vi "Post Initialize Action.vi"(8 "error in (no error)":errorcluster, 11 "Main Window in":refnum<class "Main Window.lvclass">) -> (0 "error out":errorcluster, 2 "Init Event Data":variant, 3 "Main Window out":refnum<class "Main Window.lvclass">)   [LabVIEW 2021, in "Recipe.lvlib" / "Main Window.lvclass"]
doc: "This VI is called just after the Panel Actor's UI was initialized.\n\nData wired to <b>Init Event Data</b> will be passed in the panel's \"Initialized\" user event.\n\nIf there were any initialization errors they should be handled here.\n\n----\nPlease see the following web address for additional documentation and tutorial information:\nhttp://www.mooregoodideas.com/mgi-panel-manager/\n\nAuthor: Derek Trepanier\n\nCopyright (c) 2018, Moore Good Ideas, Inc.\n\nAll rights reserved.\n\nRedistribution and use in source and binary forms, with or without modification, are permitted provided that the following conditions are met:\n\n * Redistributions of source code must retain the above copyright notice, this list of conditions and the following disclaimer.\n * Redistributions in binary form must reproduce the above copyright notice, this list of conditions and the following disclaimer in the documentation and/or other materials provided with the distribution.\n * Neither the name of Moore Good Ideas, Inc. nor the names of its contributors may be used to endorse or promote products derived from this software without specific prior written permission.\n\nTHIS SOFTWARE IS PROVIDED BY THE COPYRIGHT HOLDERS AND CONTRIBUTORS \"AS IS\" AND ANY EXPRESS OR IMPLIED WARRANTIES, INCLUDING, BUT NOT LIMITED TO, THE IMPLIED WARRANTIES OF MERCHANTABILITY AND FITNESS FOR A PARTICULAR PURPOSE ARE DISCLAIMED. IN NO EVENT SHALL THE COPYRIGHT OWNER OR CONTRIBUTORS BE LIABLE FOR ANY DIRECT, INDIRECT, INCIDENTAL, SPECIAL, EXEMPLARY, OR CONSEQUENTIAL DAMAGES (INCLUDING, BUT NOT LIMITED TO, PROCUREMENT OF SUBSTITUTE GOODS OR SERVICES; LOSS OF USE, DATA, OR PROFITS; OR BUSINESS INTERRUPTION) HOWEVER CAUSED AND ON ANY THEORY OF LIABILITY, WHETHER IN CONTRACT, STRICT LIABILITY, OR TORT (INCLUDING NEGLIGENCE OR OTHERWISE) ARISING IN ANY WAY OUT OF THE USE OF THIS SOFTWARE, EVEN IF ADVISED OF THE POSSIBILITY OF SUCH DAMAGE."
uses:
  Main Window.lvclass
  C:/Program Files (x86)/National Instruments/LabVIEW 2021/vi.lib/MGI/Panel Manager/Panel Actor/Panel Actor/Panel Actor.lvclass
  Recipe Window/Recipe Window.lvclass
  Main Window.lvclass/Main Window.ctl
  Recipe Window/Recipe Window.lvclass/Recipe Window.ctl
  <vilib>/MGI/Panel Manager/Panel/Panel/Subpanel/Subpanel.lvclass
  C:/Program Files (x86)/National Instruments/LabVIEW 2021/vi.lib/MGI/Panel Manager/Panel/Panel/Panel.lvclass
  <vilib>/MGI/Panel Manager/Panel/Panel/Subpanel/Subpanel.vi
  <vilib>/MGI/Panel Manager/Panel Actor/Panel Actor/Panel Actor.lvclass
  <vilib>/MGI/Panel Manager/Panel/Panel.lvlib
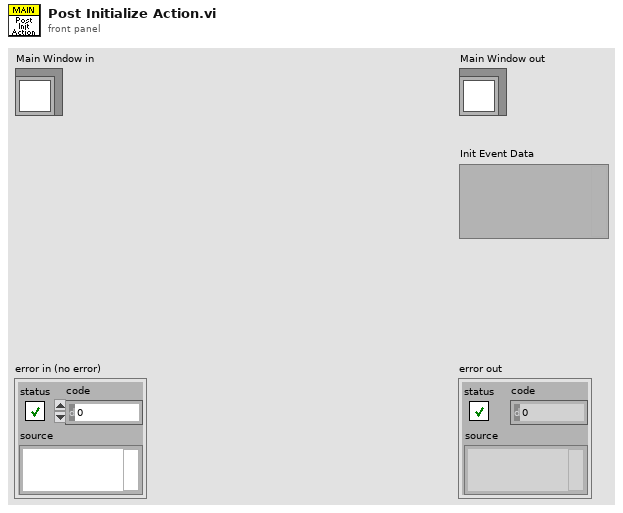
[diagram p1: front panel]
types:
  T1 = typedef "Recipe.lvlib/Main Window.lvclass/Recipe List--cluster.ctl" = T2[]
  T2 = typedef "Recipe.lvlib/Recipe Window.lvclass/Recipe Data--cluster.ctl" = cluster{"Name":string}
  T3 = map{string, refnum<class "Message Enqueuer.lvclass">}
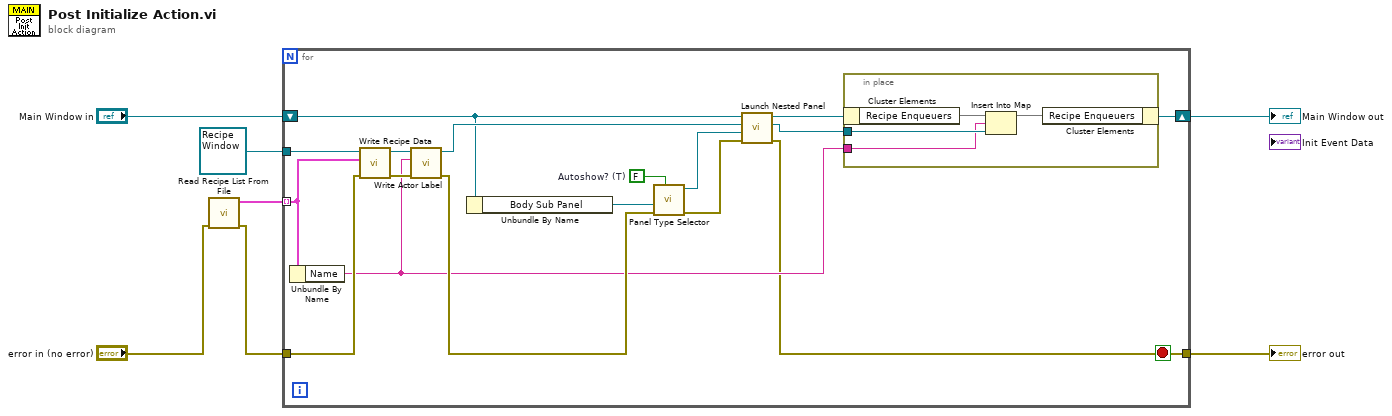
[diagram p0: block diagram]
diagram:
  n1 = call "Read Recipe List From File.vi"("error in (no error)"="error in (no error)") -> ("error out"=w6:errorcluster, "Recipe List"=w3:T1)  [unwired: 9 in]
  n2 = for {
    tunnel: w6 -> [w23]
    shift-right: [w20] -> w4
    shift-left: "Main Window in" -> [w9]
    tunnel: w3 -> [w12] mode=indexing
    tunnel: refnum<class "Recipe Window.lvclass"> refnum ("Recipe.lvlib:Recipe Window.lvclass") -> [w14]
    tunnel: [w10] -> w1
    stop <- w10 stop-if-true
    w17 = FALSE  # Autoshow? (T)
    n3 = Unbundle By Name(w12) -> ("Name"=w11:string)
    n4 = call "Write Recipe Data.vi"("error in (no error)"=w23, "Recipe Data"=w12, "Recipe Window in"=w14) -> ("error out"=w22:errorcluster, "Recipe Window out"=w13:refnum<class "Recipe Window.lvclass">)  [unwired: 7 in]
    n5 = call-dynamic "Write Actor Label.vi"("error in (no error)"=w22, "Actor Label"=w11, "Monitored Actor in"=w13) -> ("error out"=w21:errorcluster, "Monitored Actor out"=w16:refnum<class "Recipe Window.lvclass">)  [unwired: 7 in]
    n6 = Unbundle By Name(w9) -> ("Body Sub Panel"=w8:refnum<vi>)
    n7 = call-poly <vilib>:"Panel Type Selector.vi"("Autoshow? (T)"=w17, "Error In"=w21, "Sub Panel"=w8) -> ("Error Out"=w24:errorcluster, "Subpanel Out"=w15:refnum<class "Subpanel.lvclass">)  [unwired: 7 in]
    n8 = call <vilib>:"Launch Nested Panel.vi"("error in (no error)"=w24, "Panel"=w15, "Nested Panel Actor"=w16, "Panel Actor in"=w9) -> ("error out"=w10:errorcluster, "Nested Actor's Enqueuer"=w18:refnum<class "Message Enqueuer.lvclass">, "Panel Actor out"=w19:refnum<class "Main Window.lvclass">)  [unwired: 4 in, 1 out]
    n9 = in-place {
      in-place-border: w18 -> [w26]
      in-place-border: w11 -> [w25]
      n10 = in-place-cluster #1(w19) -> ("Recipe Enqueuers"=w28:T3)
      n11 = Insert Into Map(map in=w28, key=w25, value=w26) -> (map out=w27:T3)  [unwired: 2 out]
      n12 = in-place-cluster #1("Recipe Enqueuers"=w27) -> (w20:refnum<class "Main Window.lvclass">)
    }
  }
  "error out" <- w1
  "Main Window out" <- w4
